vi "new_trend.vi"(4 "T start":timestamp, 5 "SigId":u16, 6 "T final":timestamp, 7 "connection ref":T1) -> (0 "error out":errorcluster, 1 "XY Graph":cluster{timestamp[], sgl[]}, 2 "sql":string, 3 "units":string)   [LabVIEW 2010]
uses:
  <vilib>/addons/database/Connection.llb/Conn ObjectReference.ctl
  <vilib>/addons/database/_DB Variant To Data/Database Variant To Data.xnode
  <vilib>/addons/database/NI_Database_API.lvlib
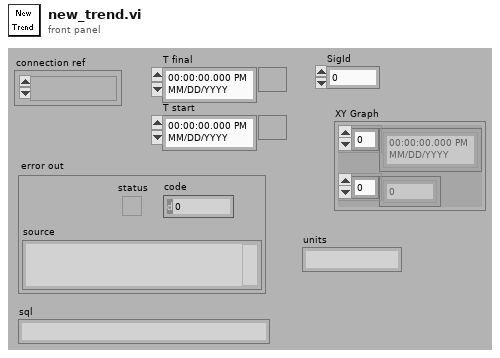
[diagram p1: front panel]
types:
  T1 = typedef "NI_Database_API.lvlib/Conn ObjectReference.ctl" = refnum<k1>
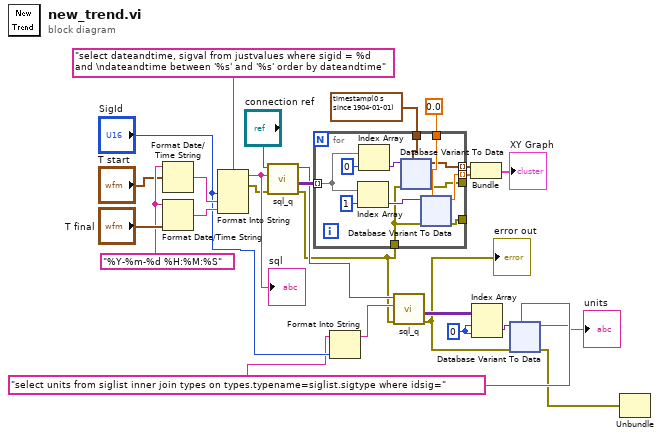
[diagram p0: block diagram]
diagram:
  w7 = 0 ("index")
  w5 = "select units from siglist inner join types on types.typename=siglist.sigtype where idsig="
  w17 = "%Y-%m-%d %H:%M:%S" ("time format string (%c)")
  n1 = Format Date/Time String(time format string (%c)=w17, seconds (now)="T start") -> (date/time string=w18:string)  [unwired: 1 in]
  n2 = Format Date/Time String(time format string (%c)=w17, seconds (now)="T final") -> (date/time string=w19:string)  [unwired: 1 in]
  n3 = Format Into String(format string="select dateandtime, sigval from justvalues where sigid = %d and \ndateandtime between '%s' and '%s' order by dateandtime" ("optional clause"), "SigId", w18, w19) -> (resulting string=w24:string, error out=w12:errorcluster)  [unwired: 2 in]
  "sql" <- w24
  n4 = call "sql_q.vi"("error in"=w12, "SQL query"=w24, "connect ref"="connection ref") -> ("error out"=w2:errorcluster, "recordset data"=w25:variant[][], "conn ref out"=w11:T1)  [unwired: 1 in, 1 out]
  n5 = for {
    tunnel: w25 -> [w30] mode=indexing
    tunnel: timestamp(0 s since 1904-01-01) ("T final") -> [w34]
    tunnel: sgl 0.0 -> [w33]
    tunnel: [w32] -> w20 mode=indexing
    tunnel: [w31] -> w21 mode=indexing
    tunnel: w2 -> [w29]
    tunnel: [w28] -> _
    tunnel: [w27] -> _
    n6 = Index Array(array=w30, index=1) -> (element=w35:variant)
    n7 = Index Array(array=w30, index=0) -> (element=w36:variant)
    n8 = xnode "Database Variant To Data"("database variant"=w36, "error in"=w29, "type"=w34) -> ("data"=w32:timestamp, "error out"=w27:errorcluster)
    n9 = xnode "Database Variant To Data"("database variant"=w35, "error in"=w29, "type"=w33) -> ("data"=w31:sgl, "error out"=w28:errorcluster)
  }
  n10 = Format Into String(initial string=w5, "SigId") -> (resulting string=w9:string)  [unwired: 2 in, 1 out]
  n11 = call "sql_q.vi"("error in"=w2, "SQL query"=w9, "connect ref"=w11) -> ("error out"=w3:errorcluster, "recordset data"=w8:variant[][])  [unwired: 1 in, 2 out]
  "error out" <- w3
  n12 = Bundle(w20, w21) -> (→"XY Graph":cluster{timestamp[], sgl[]})  [unwired: 1 in]
  n13 = Index Array(array=w8, index (row)=w7, index (col)=w7) -> (element=w6:variant)
  n14 = xnode "Database Variant To Data"("database variant"=w6, "error in"=w3, "type"=w5) -> ("data"=→"units":string, "error out"=w1:errorcluster)
  n15 = Unbundle(w1) -> ()  [unwired: 3 out]
